vi "puertayalarma.vi"() -> ()   [LabVIEW 2021]
panel:
  in  "Sensor  Proximidad 3":bool
  in  "Sensor  Proximidad 2":bool
  in  "Sensor  Proximidad 1":bool
  in  "ActAlarm":bool
  out "Sirena":bool
  out "ESTADO ALARMA":string
  out "Muestra Señal Entrada":dbl
  in  "Señal Entrada":dbl min=0.0 max=255.0 step=255.0
  out "Puerta3":bool
  out "Puerta2":bool
  in  "stop":bool
  out "Puerta1":bool
  # "PANEL PUERTAS AUTOMATICAS"
  # "PANEL DE SISTEMA SEGURIDAD"
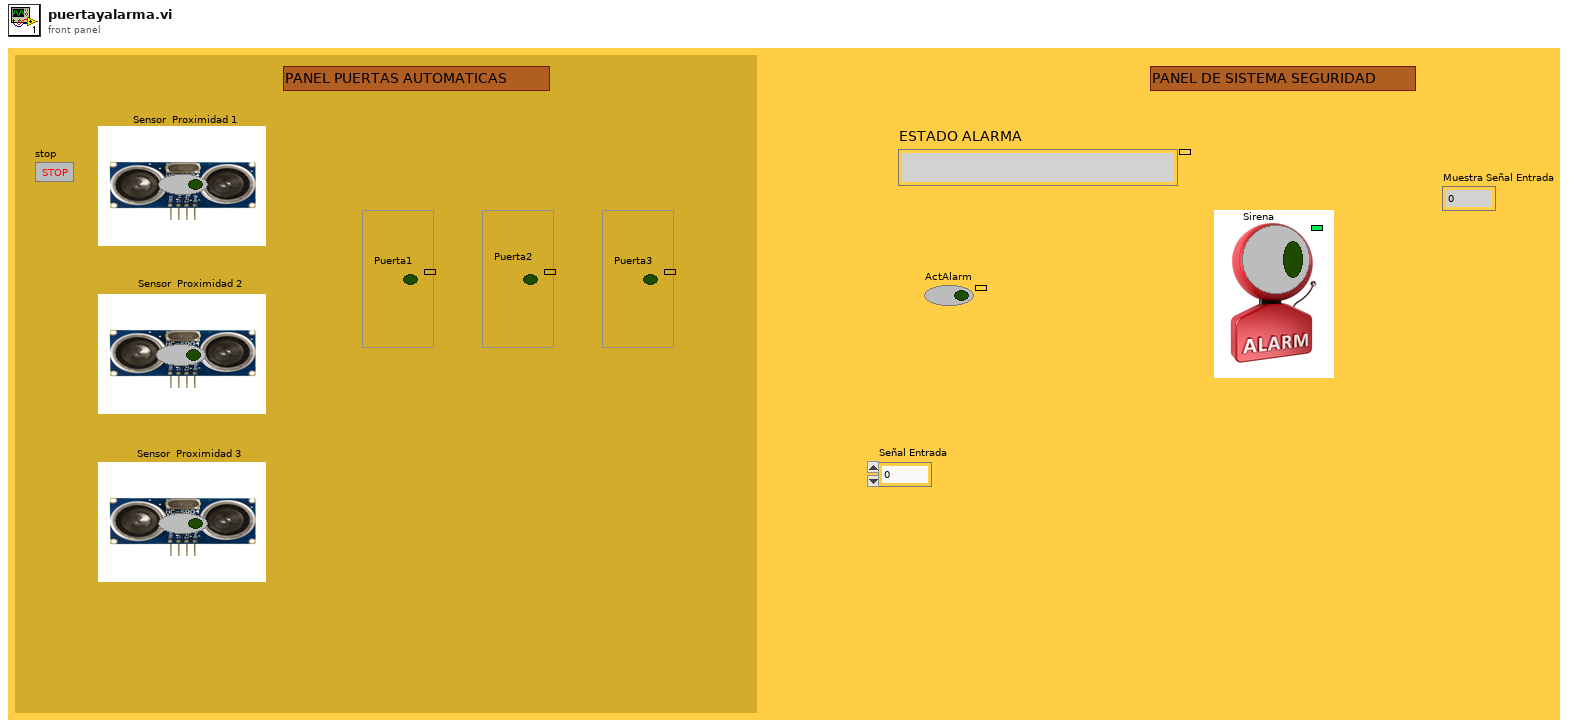
[diagram p1: front panel]
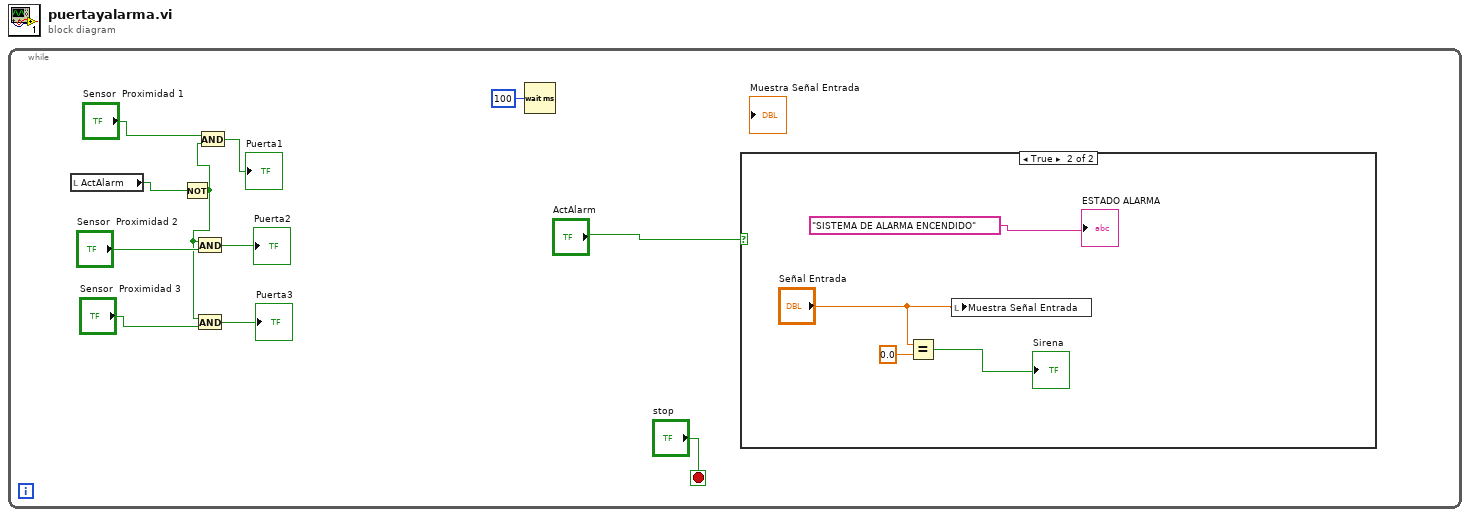
[diagram p0: block diagram]
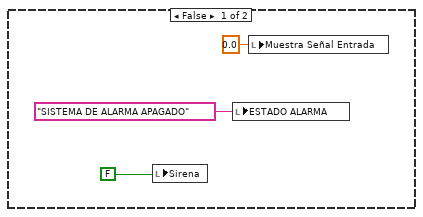
[diagram p2: hidden frame]
diagram:
  n1 = while {
    stop <- "stop" stop-if-true
    n2 = local read "ActAlarm"() -> (w8:bool)
    n3 = Not(x=w8) -> (.not. x?=w3:bool)
    n4 = And(x=w3, y="Sensor  Proximidad 2") -> (x .and. y?=→"Puerta2":bool)
    n5 = And(x=w3, y="Sensor  Proximidad 3") -> (x .and. y?=→"Puerta3":bool)
    n6 = And(x="Sensor  Proximidad 1", y=w3) -> (x .and. y?=→"Puerta1":bool)
    n7 = Wait (ms)(milliseconds to wait=u32 100) -> ()  [unwired: 1 out]
    n8 = case shown="True" "ActAlarm" {
      frame False {
        n9 = local write "Sirena"(FALSE) -> ()
        n10 = local write "ESTADO ALARMA"("SISTEMA DE ALARMA APAGADO" ("ESTADO DE ALARMA")) -> ()
        n11 = local write "Muestra Señal Entrada"(0.0 ("Muestra Señal Entrada")) -> ()
      }
      frame True {
        n12 = Equal?(x="Señal Entrada", y=0.0) -> (x = y?=→"Sirena":bool)
        n13 = local write "Muestra Señal Entrada"("Señal Entrada") -> ()
        "ESTADO ALARMA" <- "SISTEMA DE ALARMA ENCENDIDO"
      }
    }
  }
